vi "XciteCh_structure.vi"() -> (0 "XCiteCh":T1, 1 "XCiteC_raw":T2, 2 "StructSize":i32, 3 "RawStructSize":i32)   [LabVIEW 2019, in "XCite.lvlib"]
doc: "Creates a strucrure that is is used in the larger XCiteStructure. Also generates a LabVIEW-friendly version of the structure."
uses:
  XCite.lvlib
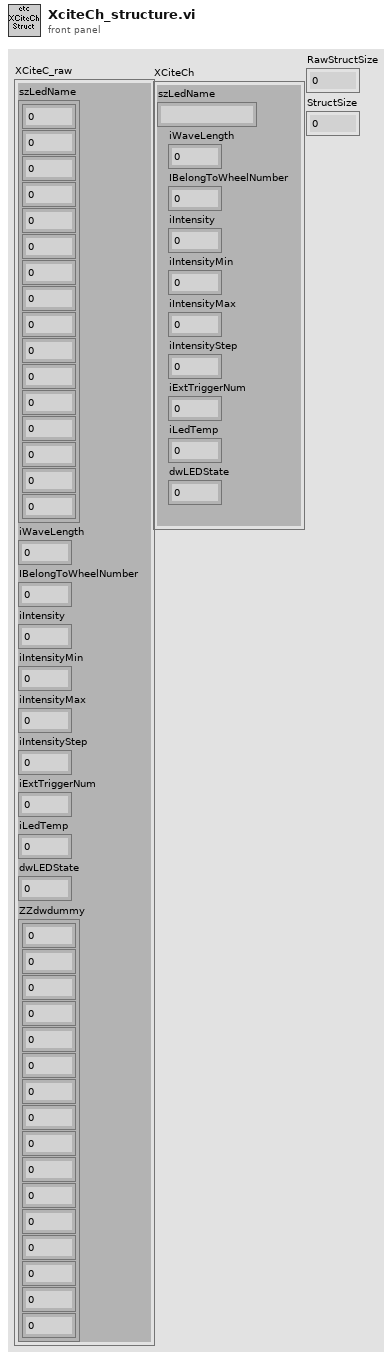
[diagram p1: front panel]
types:
  T1 = cluster{"szLedName":string, "iWaveLength":i32, "IBelongToWheelNumber":i32, "iIntensity":i32, "iIntensityMin":i32, "iIntensityMax":i32, "iIntensityStep":i32, "iExtTriggerNum":i32, "iLedTemp":i32, "dwLEDState":u32}
  T2 = cluster{"szLedName":cluster{u8, u8, u8, u8, u8, u8, u8, u8, u8, u8, u8, u8, u8, u8, u8, u8}, "iWaveLength":i32, "IBelongToWheelNumber":i32, "iIntensity":i32, "iIntensityMin":i32, "iIntensityMax":i32, "iIntensityStep":i32, "iExtTriggerNum":i32, "iLedTemp":i32, "dwLEDState":u32, "ZZdwdummy":cluster{u32, u32, u32, u32, u32, u32, u32, u32, u32, u32, u32, u32, u32, u32, u32, u32}}
  T3 = cluster{u32, u32, u32, u32, u32, u32, u32, u32, u32, u32, u32, u32, u32, u32, u32, u32}
  T4 = cluster{u8, u8, u8, u8, u8, u8, u8, u8, u8, u8, u8, u8, u8, u8, u8, u8}
  T5 = cluster{"string":string, "iWaveLength":i32, "IBelongToWheelNumber":i32, "iIntensity":i32, "iIntensityMin":i32, "iIntensityMax":i32, "iIntensityStep":i32, "iExtTriggerNum":i32, "iLedTemp":i32, "dwLEDState":u32}
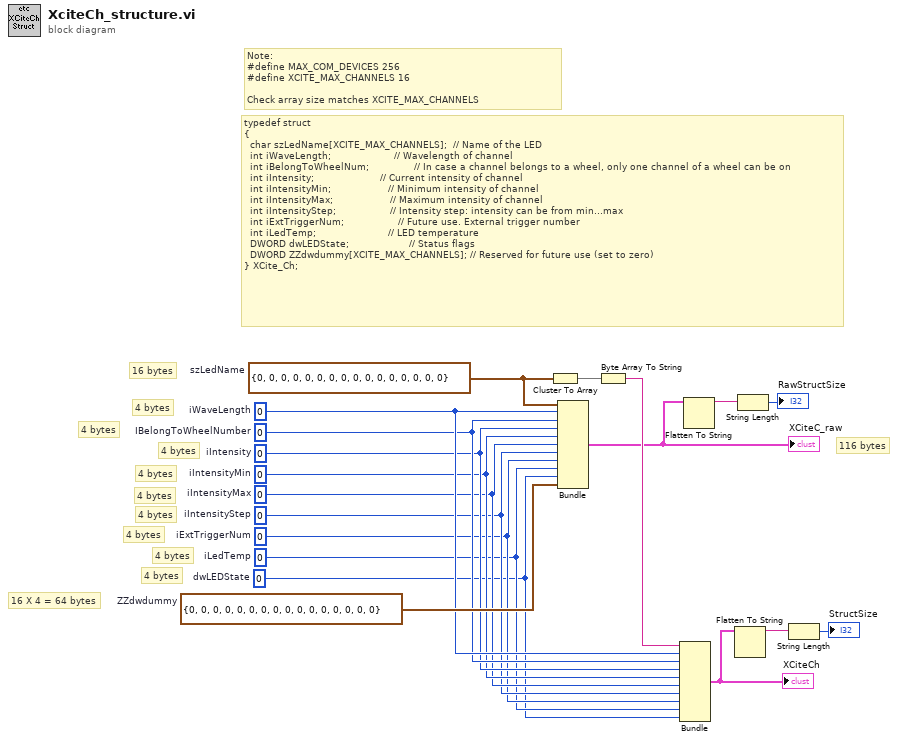
[diagram p0: block diagram]
diagram:
  w19 = T3 {0, 0, 0, 0, 0, 0, 0, 0, 0, 0, 0, 0, 0, 0, 0, 0}  # ZZdwdummy
  w7 = u32 0  # dwLEDState
  w8 = 0  # iLedTemp
  w9 = 0  # iExtTriggerNum
  w10 = 0  # iIntensityStep
  w11 = 0  # iIntensityMax
  w12 = 0  # iIntensityMin
  w13 = 0  # iIntensity
  w14 = 0  # IBelongToWheelNumber
  w15 = 0  # iWaveLength
  w18 = T4 {0, 0, 0, 0, 0, 0, 0, 0, 0, 0, 0, 0, 0, 0, 0, 0}  # szLedName
  # "116 bytes"
  # "4 bytes"
  # "16 X 4 = 64 bytes"
  # "4 bytes"
  # "4 bytes"
  # "4 bytes"
  # "4 bytes"
  # "4 bytes"
  # "4 bytes"
  # "4 bytes"
  # "4 bytes"
  # "16 bytes"
  # "Note:\n#define MAX_COM_DEVICES 256\n#define XCITE_MAX_CHANNELS 16\n\nCheck array size matches XCITE_MAX_CHANNELS"
  # "typedef struct\n{\n  char szLedName[XCITE_MAX_CHANNELS];  // Name of the LED\n  int iWaveLength;                     // Wavelength of channel\n  int iBelongToWheelNum;               // In case a channel belongs to a wheel, only one channel of a wheel can be on\n  int iIntensity;                      // Current intensity of channel\n  int iIntensityMin;                   // Minimum intensity of channel\n  int iIntensityMax;                   // Maximum intensity of channel\n  int iIntensityStep;                  // Intensity step: intensity can be from min...max\n  int iExtTriggerNum;                  // Future use. External trigger number\n  int iLedTemp;                        // LED temperature\n  DWORD dwLEDState;                    // Status flags\n  DWORD ZZdwdummy[XCITE_MAX_CHANNELS]; // Reserved for future use (set to zero)\n} XCite_Ch;"
  n1 = Cluster To Array(cluster=w18) -> (array=w17:u8[])
  n2 = Bundle("szLedName"=w18, "iWaveLength"=w15, "IBelongToWheelNumber"=w14, "iIntensity"=w13, "iIntensityMin"=w12, "iIntensityMax"=w11, "iIntensityStep"=w10, "iExtTriggerNum"=w9, "iLedTemp"=w8, "dwLEDState"=w7, "ZZdwdummy"=w19) -> (w4:T2)  [unwired: 1 in]
  "XCiteC_raw" <- w4
  n3 = Byte Array To String(unsigned byte array=w17) -> (string=w16:string)
  n4 = Bundle("string"=w16, "iWaveLength"=w15, "IBelongToWheelNumber"=w14, "iIntensity"=w13, "iIntensityMin"=w12, "iIntensityMax"=w11, "iIntensityStep"=w10, "iExtTriggerNum"=w9, "iLedTemp"=w8, "dwLEDState"=w7) -> (w3:T5)  [unwired: 1 in]
  "XCiteCh" <- w3
  n5 = Flatten To String(anything=w4) -> (data string=w6:string)  [unwired: 3 in, 2 out]
  n6 = Flatten To String(anything=w3) -> (data string=w5:string)  [unwired: 3 in, 2 out]
  n7 = String Length(string=w6) -> (length=→"RawStructSize":i32)
  n8 = String Length(string=w5) -> (length=→"StructSize":i32)
